vi "timezone_temporary.vi"() -> ()   [LabVIEW 2013]
panel:
  out "Array 3":string[](array[string])
  out "Minutes":i32[](array[numeric])
  in  "Input Vector":timestamp[](array[timestamp])=[timestamp(3792895200 s since 1904-01-01), timestamp(3792897000 s since 1904-01-01), timestamp(3792898740 s since 1904-01-01), timestamp(3792898800 s since 1904-01-01), timestamp(3792898860 s since 1904-01-01), timestamp(3792902340 s since 1904-01-01), timestamp(3813454740 s since 1904-01-01), timestamp(3813458400 s since 1904-01-01), timestamp(3813460200 s since 1904-01-01), timestamp(3813461940 s since 1904-01-01), timestamp(3813462000 s since 1904-01-01), timestamp(3813463800 s since 1904-01-01), timestamp(3813465540 s since 1904-01-01), timestamp(3818449906.6740217 s since 1904-01-01), timestamp(3810988740 s since 1904-01-01), timestamp(3810988800 s since 1904-01-01), timestamp(3795263940 s since 1904-01-01), timestamp(3795264000 s since 1904-01-01), timestamp(3794691540 s since 1904-01-01), timestamp(3794691600 s since 1904-01-01), timestamp(3812831940 s since 1904-01-01), timestamp(3812835600 s since 1904-01-01), timestamp(3792898740 s since 1904-01-01), timestamp(3792898800 s since 1904-01-01), timestamp(3844907940 s since 1904-01-01), timestamp(3844915200 s since 1904-01-01), timestamp(3811057140 s since 1904-01-01), timestamp(3811082340 s since 1904-01-01), timestamp(3811111140 s since 1904-01-01)] format="%<%.3X %x>T"
  out "Hours":i32[](array[numeric])
  # "AUS +10:00\n||\n||\nAUS +11:00\n||\n||\nAUS +10:00"
  # "Paris +01:00\n||\n||\nParis +02:00\n||\n||\nParis +01:00"
  # "USA East -05:00\n||\n||\nUSA East -04:00\n||\n||\nUSA East -05:00"
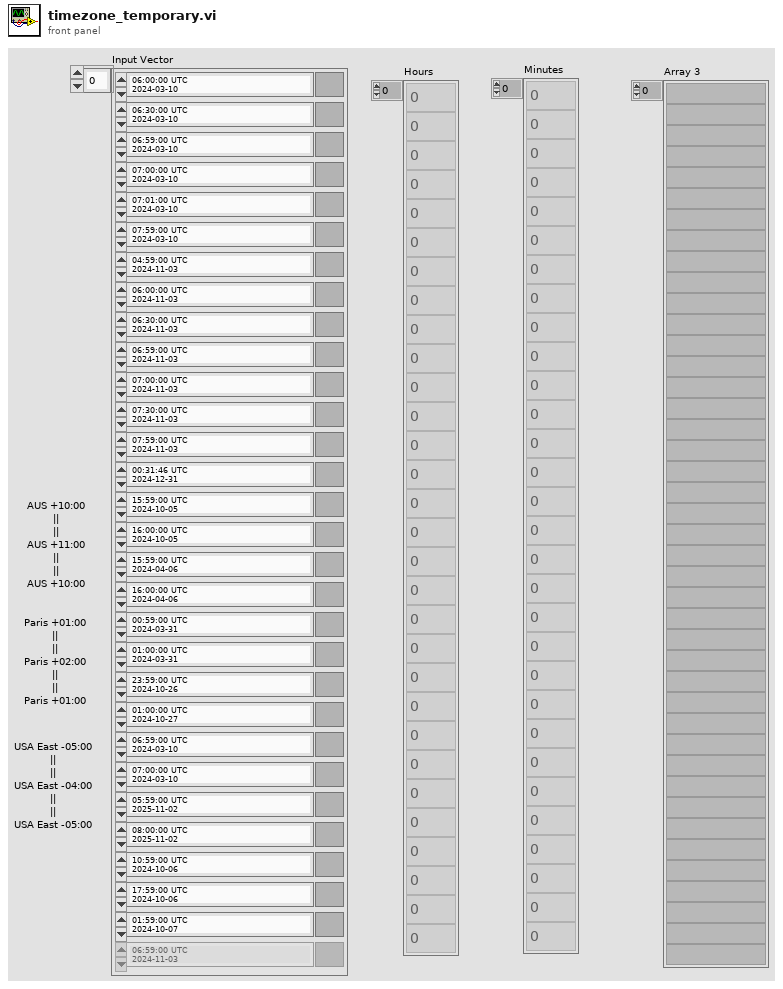
[diagram p1: front panel]
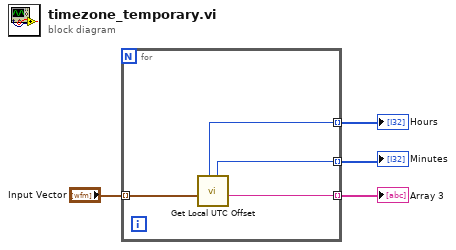
[diagram p0: block diagram]
diagram:
  n1 = for {
    tunnel: "Input Vector" -> [w8] mode=indexing
    tunnel: [w5] -> w4 mode=indexing
    tunnel: [w6] -> w2 mode=indexing
    tunnel: [w7] -> w1 mode=indexing
    n2 = call "Get Local UTC Offset.vi"("timestamp (now)"=w8) -> ("UTC Offset String"=w7:string, "UTC Offset (minutes)"=w6:i32, "UTC Offset (hours)"=w5:i32)  [unwired: 7 in, 1 out]
  }
  "Hours" <- w4
  "Minutes" <- w2
  "Array 3" <- w1
